vi "Menu_Invoke Node.vi"(11 "Affected Items Out":T1) -> (3 "Menu Items To Add":T2(array[cluster]))   [LabVIEW 2023]
uses:
  top/BundleMagic.ctl
  controls/action enum.ctl
panel:
  out "Enabled Status":enum8{"Enabled", "Disabled"}[](array[ring])
  out "Menu Item Display Name":string[](array[string])
  out "Position In Menu":T3(array[cluster])
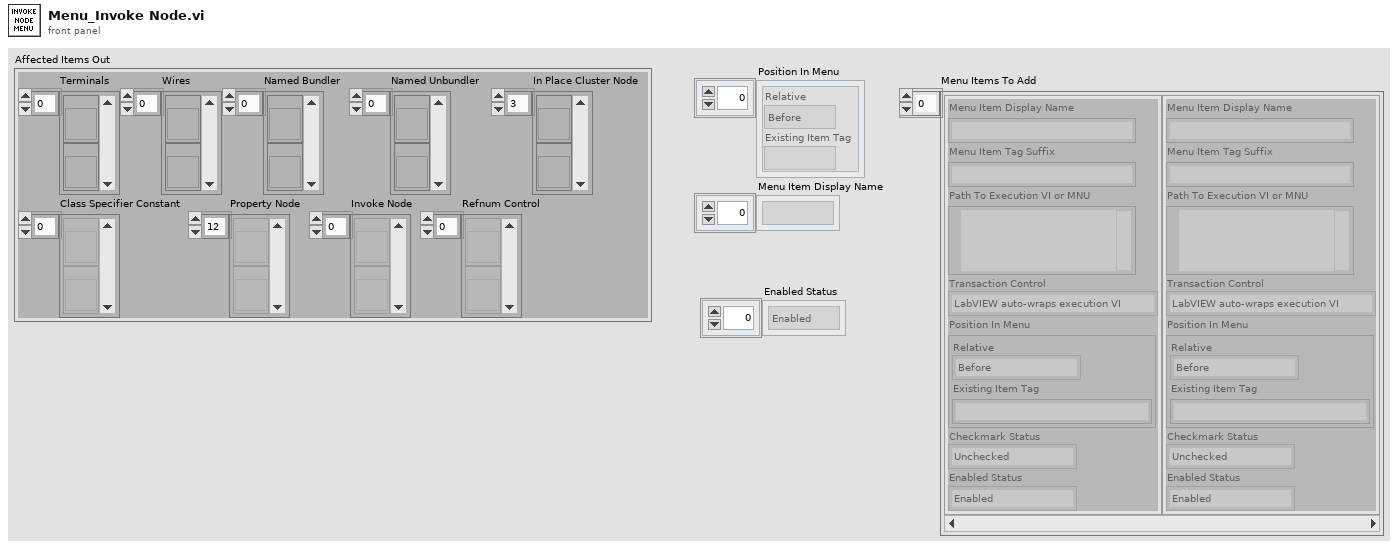
[diagram p1: front panel]
types:
  T1 = typedef "BundleMagic.ctl" = cluster{"Terminals":refnum<vi>[], "Wires":refnum<vi>[], "Named Bundler":refnum<vi>[], "Named Unbundler":refnum<vi>[], "In Place Cluster Node":refnum<vi>[], "Class Specifier Constant":refnum<vi>[], "Property Node":refnum<vi>[], "Invoke Node":refnum<vi>[], "Refnum Control":refnum<vi>[]}
  T2 = cluster{"Menu Item Display Name":string, "Menu Item Tag Suffix":string, "Path To Execution VI or MNU":path, "Transaction Control":enum8{"LabVIEW auto-wraps execution VI", "Execution VI will define if needed"}, "Position In Menu":cluster{"Relative":enum8{"Before", "Instead of", "After", "Into Submenu"}, "Existing Item Tag":string}, "Checkmark Status":enum8{"Unchecked", "Checked"}, "Enabled Status":enum8{"Enabled", "Disabled"}}[]
  T3 = cluster{"Relative":enum8{"Before", "Instead of", "After", "Into Submenu"}, "Existing Item Tag":string}[]
  T4 = typedef "action enum.ctl" = enum16{"[NONE]", "APP_SEPARATOR", "Wire Bundle", "Wire Unbundle", "Terminal Unbundle", "Terminal Bundle", "Bundler Move Up", "Bundler Move Down", "Bundler Insert", "Bundler Remove", "Bundler Remove Unwired", "Bundler Rearrange", "In Place Insert", "In Place Remove", "In Place Remove Unwired", "In Place Rearrange", "Wire Properties", "Wire Method", "Terminal Properties", "Terminal Method", "Property Move Up", "Property Move Down", "Properties Insert", "Properties Remove", "Properties Remove Unwired", "Properties Rearrange", "Method Change", "Class For Constant", "Class For Control", "Class For Node", "Class Name to Clipboard"}
  T5 = cluster{"Menu Item Display Name":string, "Menu Item Tag Suffix":string, "Path To Execution VI or MNU":path, "Transaction Control":enum8{"LabVIEW auto-wraps execution VI", "Execution VI will define if needed"}, "Position In Menu":cluster{"Relative":enum8{"Before", "Instead of", "After", "Into Submenu"}, "Existing Item Tag":string}, "Checkmark Status":enum8{"Unchecked", "Checked"}, "Enabled Status":enum8{"Enabled", "Disabled"}}
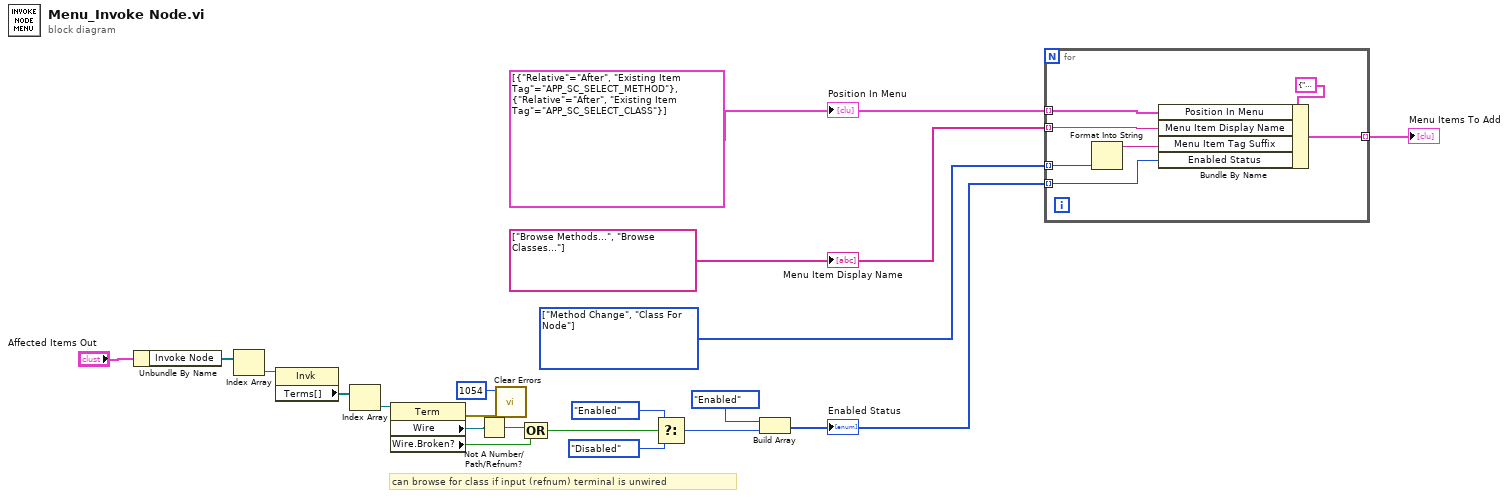
[diagram p0: block diagram]
diagram:
  w1 = T4[] [enum."Method Change", enum."Class For Node"] items=["[NONE]", "APP_SEPARATOR", "Wire Bundle", "Wire Unbundle", "Terminal Unbundle", "Terminal Bundle", "Bundler Move Up", "Bundler Move Down", "Bundler Insert", "Bundler Remove", "Bundler Remove Unwired", "Bundler Rearrange", "In Place Insert", "In Place Remove", "In Place Remove Unwired", "In Place Rearrange", "Wire Properties", "Wire Method", "Terminal Properties", "Terminal Method", "Property Move Up", "Property Move Down", "Properties Insert", "Properties Remove", "Properties Remove Unwired", "Properties Rearrange", "Method Change", "Class For Constant", "Class For Control", "Class For Node", "Class Name to Clipboard"] ("Array")
  w20 = T3 [{"Relative"=enum."After", "Existing Item Tag"="APP_SC_SELECT_METHOD"}, {"Relative"=enum."After", "Existing Item Tag"="APP_SC_SELECT_CLASS"}]
  w19 = string[] ["Browse Methods...", "Browse Classes..."]
  # "can browse for class if input (refnum) terminal is unwired"
  n1 = Unbundle By Name("Affected Items Out") -> ("Invoke Node"=w17:refnum<vi>[])
  n2 = Index Array(array=w17) -> (element=w12:refnum<vi>)  [unwired: 1 in]
  n3 = property class="Invk"(reference=w12) -> ("Terms[]"=w5:refnum<vi>[])  [unwired: 1 in, 2 out]
  n4 = Index Array(array=w5) -> (element=w16:refnum<vi>)  [unwired: 1 in]
  n5 = property class="Term"(reference=w16) -> (error out=w8:errorcluster, "Wire"=w15:refnum<vi>, "Wire.Broken?"=w11:bool)  [unwired: 1 in, 1 out]
  n6 = Not A Number/Path/Refnum?(number/path/refnum=w15) -> (NaN/Path/Refnum?=w10:bool)
  n7 = call <vilib>:"Clear Errors.vi"("error in (no error)"=w8, "specific error code to clear (0: all)"=1054) -> ()  [unwired: 4 in, 2 out]
  n8 = Compound Arithmetic op=OR(w10, w11) -> (w9:bool)
  n9 = Select(t=enum8{"Enabled", "Disabled"}."Enabled" ("Enabled Status"), s=w9, f=enum8{"Enabled", "Disabled"}."Disabled" ("Enabled Status")) -> (s? t:f=w3:enum8{"Enabled", "Disabled"})
  n10 = Build Array(enum8{"Enabled", "Disabled"}."Enabled" ("Enabled Status"), w3) -> (w2:enum8{"Enabled", "Disabled"}[])
  "Enabled Status" <- w2
  n11 = for {
    tunnel: [w27] -> w18 mode=indexing
    tunnel: w19 -> [w26] mode=indexing
    tunnel: w1 -> [w21] mode=indexing
    tunnel: w20 -> [w24] mode=indexing
    tunnel: w2 -> [w23] mode=indexing
    n12 = Format Into String(w21) -> (resulting string=w22:string)  [unwired: 3 in, 1 out]
    n13 = Bundle By Name(cluster=T5 {"Menu Item Display Name"="", "Menu Item Tag Suffix"="", "Path To Execution VI or MNU"=path "", "Transaction Control"=enum."LabVIEW auto-wraps execution VI", "Position In Menu"={"Relative"=enum."Before", "Existing Item Tag"=""}, "Checkmark Status"=enum."Unchecked", "Enabled Status"=enum."Enabled"} ("Cluster"), "Position In Menu"=w24, "Menu Item Display Name"=w26, "Menu Item Tag Suffix"=w22, "Enabled Status"=w23) -> (w27:T5)
  }
  "Menu Items To Add" <- w18
  "Position In Menu" <- w20
  "Menu Item Display Name" <- w19
